vi "ToString.vi"(8 "error in (no error)":errorcluster, 11 "Floating point base in":refnum<class "Floating point base.lvclass">) -> (0 "error out":errorcluster, 2 "String":string, 3 "Floating point base out":refnum<class "Floating point base.lvclass">)   [LabVIEW 2018, in "D Datagrid Library.lvlib" / "Floating point base.lvclass"]
uses:
  Floating point base.lvclass
  DatagridElement/DatagridElement.lvclass
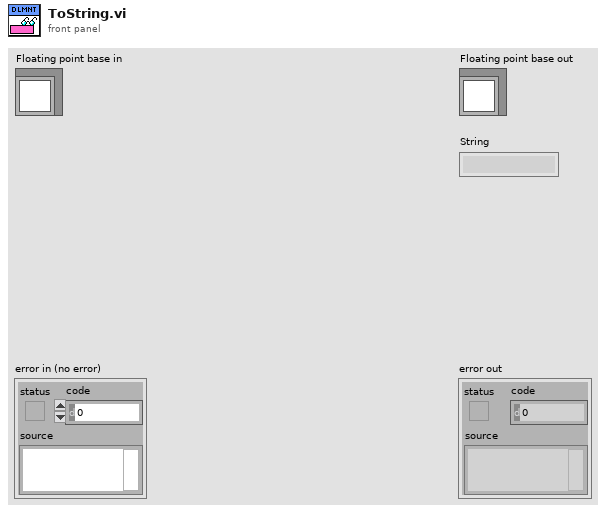
[diagram p1: front panel]
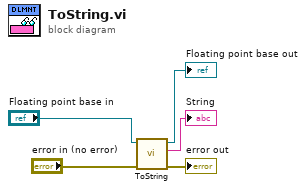
[diagram p0: block diagram]
diagram:
  n1 = call-parent "ToString.vi"("error in (no error)"="error in (no error)", "DatagridElement in"="Floating point base in") -> ("error out"=→"error out":errorcluster, "String"=→"String":string, "DatagridElement out"=→"Floating point base out":refnum<class "Floating point base.lvclass">)  [unwired: 7 in]
